vi "ProdaNG.LogOut.vi"(8 "error in":errorcluster, 11 "dbHandleIn":i32) -> (0 "error out":errorcluster)   [LabVIEW 2016]
doc: "The function allows the Logoff from the Oracle database. A return value passes back the result of the termination of the connection. It can be called in every thread. The connection to ORACLE is being terminated for the context of the specified Handle and all resources of the handle will be released. If it is being worked with a Shared Context, no thread can access ORACLE afterwards!\n\nParameter:\nHandle is invalid when it is being returned from the function and must not be used!\n\nReturncodes:\n0 no Error\n< 0 ORACLE Error code. Because the Handle is invalid when returning from the function, the function GetLastErrorMsg() cannot be used.\n6 (ERROR_INVALID_HANDLE) in case of an invalid handle"
uses:
  prodllNG.dll
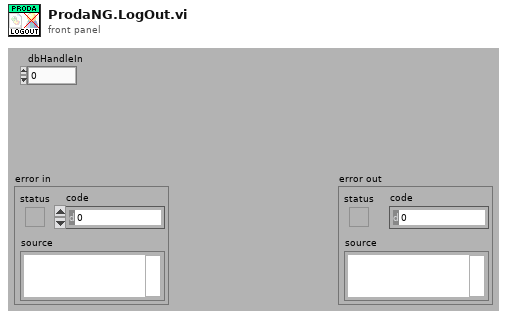
[diagram p1: front panel]
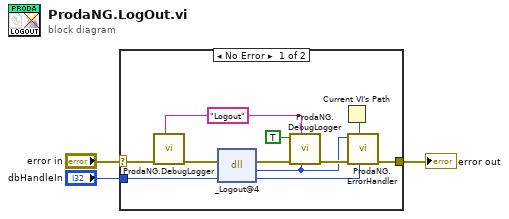
[diagram p0: block diagram]
diagram:
  n1 = case shown="No Error" "error in" {
    selector: "error in" -> [w8 w14]
    tunnel: [w13 w14] -> w2
    tunnel: "dbHandleIn" -> [w11 _]
    frame No Error {
      w10 = "Logout" ("cmd")
      n2 = call "ProdaNG.DebugLogger.vi"("cmd"=w10, "error in (no error)"=w8) -> ("error out"=w7:errorcluster)  [unwired: 9 in]
      n3 = dll-call lib="D:/svn/LineTraceSystem/SOFTWARE/sources/Database/ProdaNG/prodllNG.dll" fn="_Logout@4" ("ProDll.dll:Login")(error in=w7, "dbHandle"=w11) -> (error out=w6:errorcluster, w4:i32)  [unwired: 3 in, 1 out]
      n4 = call "ProdaNG.DebugLogger.vi"("return type"=w4, "cmd"=w10, "error in (no error)"=w6, "done? (F)"=TRUE) -> ("error out"=w5:errorcluster)  [unwired: 7 in]
      n5 = Current VI's Path() -> (path=w12:path)
      n6 = call "ProdaNG.ErrorHandler.vi"("dbHandleIn"=w11, "Path"=w12, "error in"=w5, "output_parameter"=w4) -> ("error out"=w13:errorcluster)  [unwired: 7 in]
    }
    frame Error {
    }
  }
  "error out" <- w2
